vi "library_variable.vi"() -> ()   [LabVIEW 2020, in "queue_core_loop.lvlib"]
uses:
  queue_core_loop.lvlib
  PTRL/dev_and_debug_tools/QueueMessage typedef.ctl
  PTRL/dev_and_debug_tools/dev_and_debug_tools.lvlib
panel:
  in  "ALA_Display_Queue ref":refnum<queue>
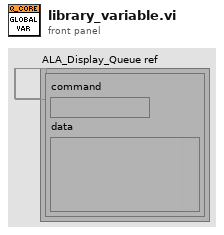
[diagram p1: front panel]
diagram:
